vi "Copy Scripting API to Installed Location.vi"(5 "Files Generated by Build":path[](array[path]), 6 "Top Level/Always Included VIs":path[](array[path]), 7 "Destination Path":path, 8 "error in (no error)":errorcluster, 9 "Target Name":string, 10 "Build Specification Name":string, 11 "Project Path":path) -> (0 "error out":errorcluster)   [LabVIEW 2017, in "Build VIs.lvlib"]
doc: "This VI is called after each run of a build specification. The VI will copy the generated LLB (Engine or System Explorer) into the VeriStand Custom Device folder (...\\Documents\\National Instruments\\NI VeriStand 2013...)."
uses:
  Build VIs.lvlib
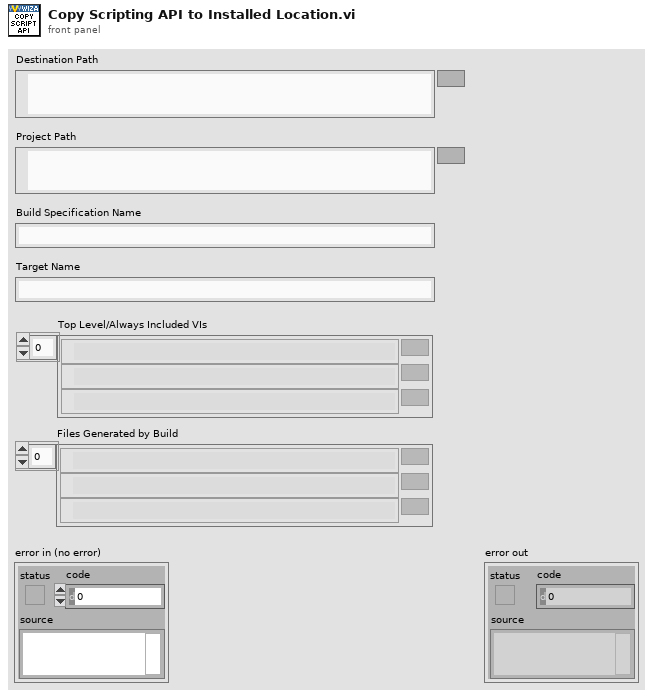
[diagram p1: front panel]
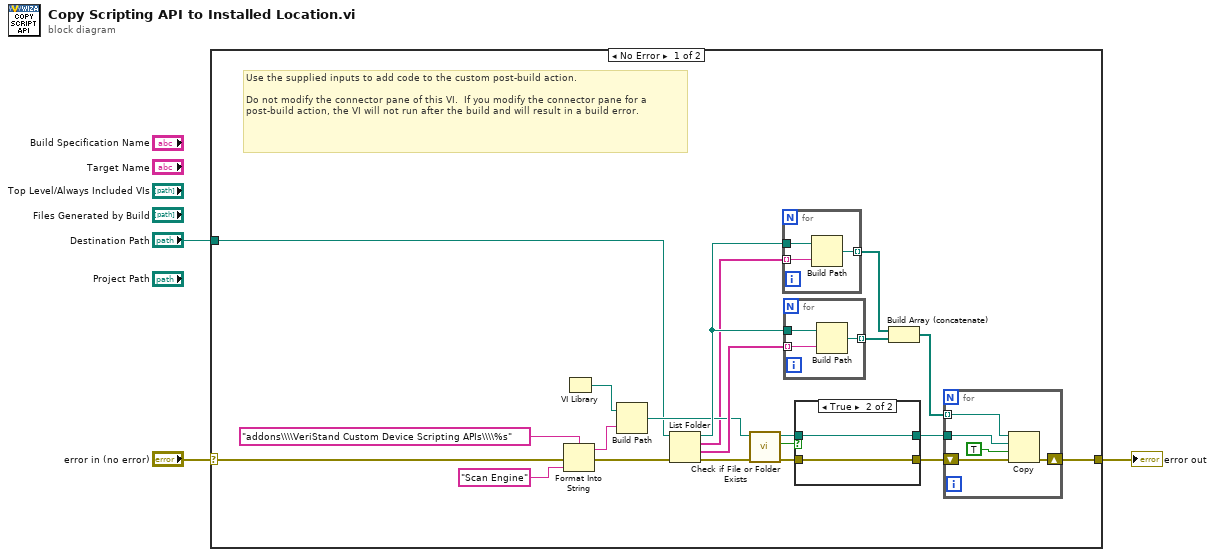
[diagram p0: block diagram]
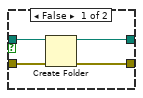
[diagram p2: hidden frame]
diagram:
  n1 = case shown="No Error" "error in (no error)" {
    selector: "error in (no error)" -> [w24 w42]
    tunnel: [w23 w42] -> w2
    tunnel: "Destination Path" -> [w5 _]
    frame No Error {
      # "Use the supplied inputs to add code to the custom post-build action.\n\nDo not modify the connector pane of this VI.  If you modify the connector pane for a post-build action, the VI will not run after the build and will result in a build error."
      n2 = Format Into String(format string="addons\\\\VeriStand Custom Device Scripting APIs\\\\%s" ("name or relative path"), error in=w24, "Scan Engine" ("CD Name")) -> (resulting string=w13:string, error out=w10:errorcluster)  [unwired: 1 in]
      n3 = VI Library() -> (path=w6:path)
      n4 = Build Path(base path=w6, name or relative path=w13) -> (appended path=w11:path)
      n5 = List Folder(path=w5, error in=w10) -> (path out=w16:path, filenames=w8:string[], folder names=w17:string[], error out=w14:errorcluster)  [unwired: 2 in]
      n6 = call <vilib>:"Check if File or Folder Exists.vi"("error in (no error)"=w14, "path"=w11) -> ("error out"=w18:errorcluster, "file or folder exists?"=w20:bool, "dup path"=w19:path)  [unwired: 7 in]
      n7 = for {
        tunnel: w8 -> [w40] mode=indexing
        tunnel: w16 -> [w41]
        tunnel: [w39] -> w22 mode=indexing
        n8 = Build Path(base path=w41, name or relative path=w40) -> (appended path=w39:path)
      }
      n9 = for {
        tunnel: w17 -> [w37] mode=indexing
        tunnel: w16 -> [w38]
        tunnel: [w36] -> w15 mode=indexing
        n10 = Build Path(base path=w38, name or relative path=w37) -> (appended path=w36:path)
      }
      n11 = case shown="True" w20 {
        tunnel: w19 -> [w28 w30]
        tunnel: w18 -> [w27 w29]
        tunnel: [w26 w30] -> w7
        tunnel: [w25 w29] -> w9
        frame False {
          n12 = Create Folder(path (use dialog)=w28, error in=w27) -> (created path=w26:path, error out=w25:errorcluster)  [unwired: 1 in, 1 out]
        }
        frame True {
        }
      }
      n13 = Build Array (concatenate)(w22, w15) -> (w21:path[])
      n14 = for {
        tunnel: w21 -> [w32] mode=indexing
        shift-right: [w33] -> w23
        shift-left: w9 -> [w34]
        tunnel: w7 -> [w31]
        n15 = Copy(8:w34, 9:TRUE ("overwrite (F)"), 10:w31, 11:w32) -> (0:w33:errorcluster)  [unwired: 1 in, 2 out]
      }
    }
    frame Error {
    }
  }
  "error out" <- w2
